vi "串口采集电压.vi"() -> ()   [LabVIEW 2018]
uses:
  <vilib>/Instr/_visa.llb/VISA Configure Serial Port (Instr).vi
panel:
  in  "波特率":u64(ring) items=["4800", "9600", "115200"]
  out "总接收":i32[][](array[numeric])
  in  "启动":bool
  in  "基路径":path
  in  "Save":bool
  out "单次接收":u8[](array[numeric])
  out "电压":string
  in  "stop bits (10: 1 bit)":u16(ring)=10 caption="停止位（10: 1位）" items=["1.0"=10, "1.5"=15, "2.0"=20]
  in  "parity (0:none)":enum16{"None", "Odd", "Even", "Mark", "Space"}(ring) caption="奇偶（0:无）"
  in  "data bits (8)":u16=8 caption="数据比特(8)" min=5 max=8 step=1
  in  "VISA resource name":refnum<visa-resource-name> caption="VISA资源名称"
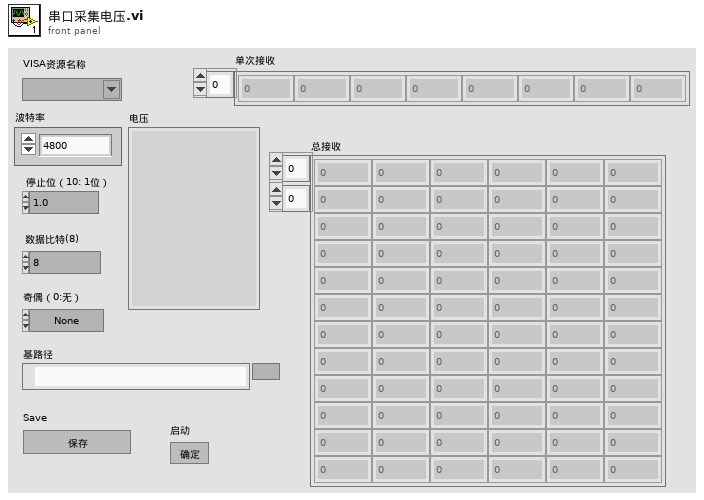
[diagram p1: front panel]
types:
  T1 = enum16{"open", "replace", "create", "open or create", "replace or create", "replace or create with confirmation"}
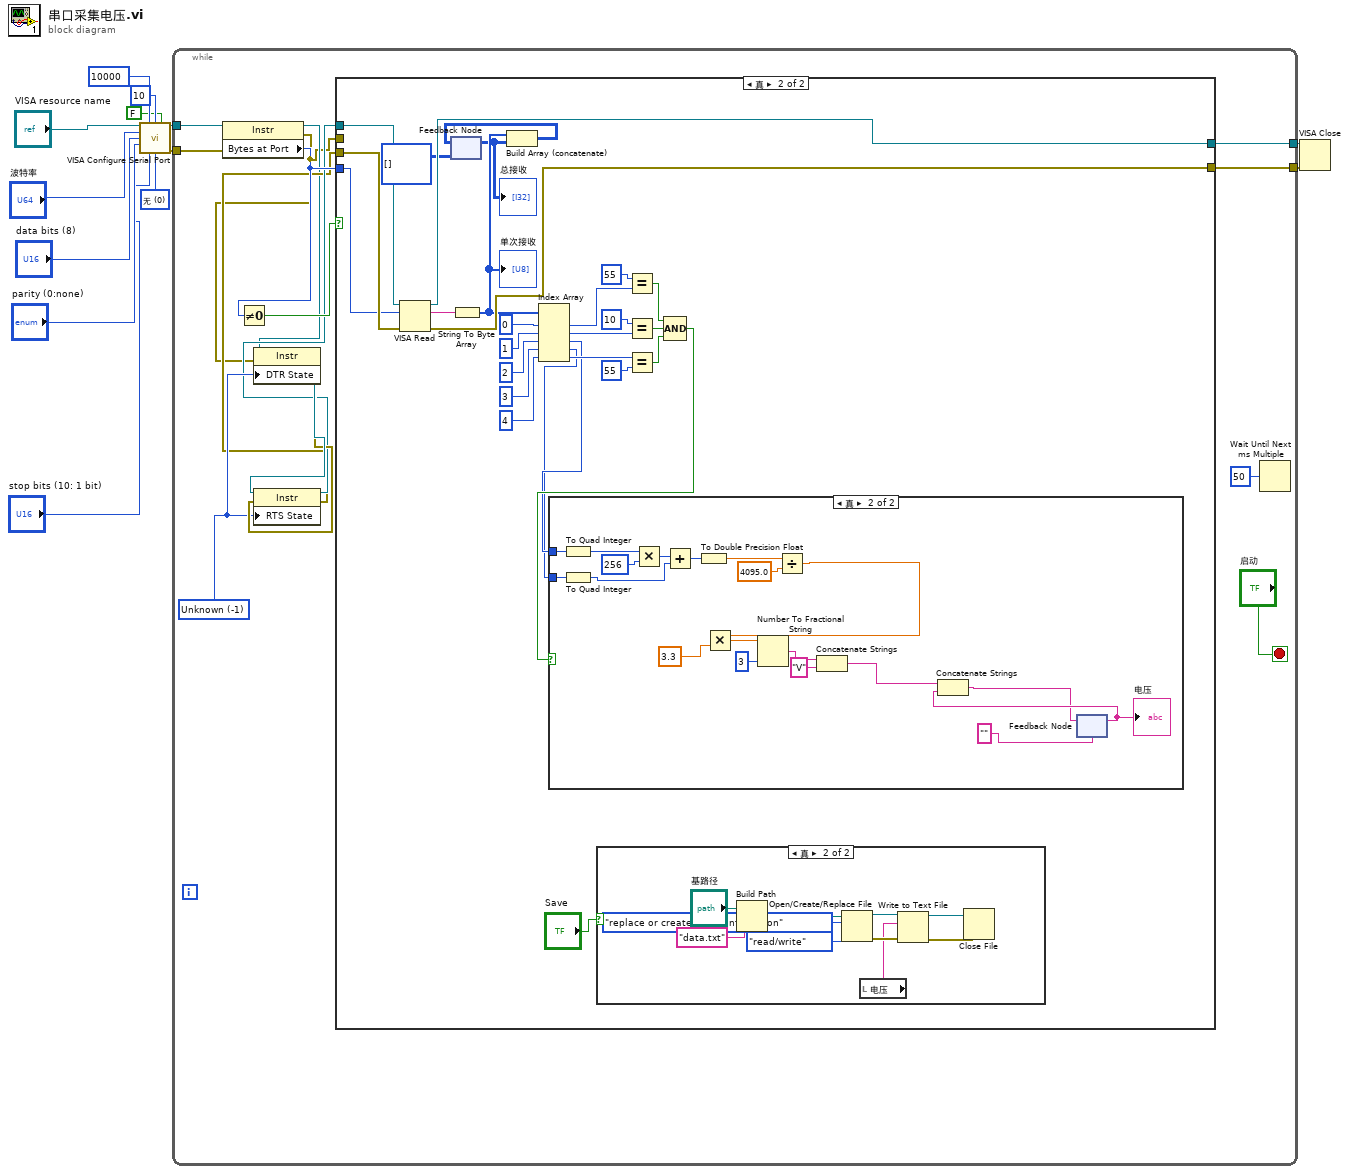
[diagram p0: block diagram]
diagram:
  w9 = u16 0 items=["无", "XON/XOFF", "RTS/CTS", "XON/XOFF & RTS/CTS", "DTR/DSR", "XON/XOFF & DTR/DSR"] ("flow control (0:none)")
  n1 = call-poly "VISA Configure Serial Port"("VISA resource name"="VISA resource name", "timeout (10sec)"=u32 10000, "termination char\n(0xA = '\\n' = LF)"=u8 10 ("termination char\n(0xA = '\\n' = LF)"), "Enable Termination\nChar (T)"=FALSE ("Enable Termination\nChar (T)"), "baud rate (9600)"="波特率", "data bits (8)"="data bits (8)", "parity (0:none)"="parity (0:none)", "stop bits (10: 1 bit)"="stop bits (10: 1 bit)", "flow control (0:none)"=w9) -> ("VISA resource name out"=w5:refnum<visa-resource-name>, "error out"=w4:errorcluster)  [unwired: 5 in]
  n2 = while {
    tunnel: w5 -> [w28]
    tunnel: w4 -> [w27]
    tunnel: [w24] -> w3
    tunnel: [w23] -> w2
    stop <- "启动" stop-if-true
    w18 = i16 -1 items=["Unknown"=-1, "Unasserted"=0, "Asserted"=1] ("Serial Settings:Modem Line Settings:Line DTR State")
    n3 = property class="Instr"(reference=w28, error in=w27) -> (reference out=w15:refnum<visa-resource-name>, error out=w14:errorcluster, "Bytes at Port"=w25:u32)
    n4 = Not Equal To 0?(x=w25) -> (x != 0?=w26:bool)
    n5 = property class="Instr"(reference=w15, error in=w14, "DTR State"=w18) -> (reference out=w20:refnum<visa-resource-name>, error out=w19:errorcluster)
    n6 = property class="Instr"(reference=w20, error in=w19, "RTS State"=w18) -> (reference out=w17:refnum<visa-resource-name>, error out=w16:errorcluster)
    n7 = case shown="真" w26 {
      tunnel: w17 -> [_ w56]
      tunnel: w16 -> [_ w55]
      tunnel: w25 -> [_ w54]
      tunnel: [_ w53] -> w24
      tunnel: [_ w52] -> w23
      tunnel: w14 -> [_ _]
      frame False {
      }
      frame True {
        n8 = VISA Read(VISA resource name=w56, byte count=w54, error in (no error)=w55) -> (VISA resource name out=w53:refnum<visa-resource-name>, read buffer=w49:string, error out=w52:errorcluster)  [unwired: 1 out]
        n9 = feedback #1(i32[][] []) -> (w44:i32[][])
        "总接收" <- w44
        n10 = String To Byte Array(string=w49) -> (unsigned byte array=w45:u8[])
        "单次接收" <- w45
        n11 = Build Array (concatenate)(w45, w44) -> (w46:i32[][])
        n12 = feedback-in #1(w46) -> ()
        n13 = Index Array(array=w45, index #1=0 ("索引"), index #2=1 ("索引"), index #3=2 ("索引"), index #4=3 ("索引"), index #5=4 ("索引")) -> (element #1=w42:u8, element #2=w40:u8, element #3=w31:u8, element #4=w30:u8, element #5=w32:u8)
        n14 = case shown="真" "Save" {
          frame False {
          }
          frame True {
            n15 = Build Path(base path="基路径", name or relative path="data.txt" ("名称或相对路径")) -> (appended path=w64:path)
            n16 = Open/Create/Replace File(file path (use dialog)=w64, operation (0:open)=T1."replace or create with confirmation" ("操作(0:open)"), access (0:read/write)=enum16{"read/write", "read-only", "write-only"}."read/write" ("权限(0:read/write)")) -> (refnum out=w61:refnum<file>, error out=w60:errorcluster)  [unwired: 3 in, 1 out]
            n17 = local read "电压"() -> (w57:string)
            n18 = Write to Text File(file (use dialog)=w61, text=w57, error in=w60) -> (refnum out=w59:refnum<file>, error out=w58:errorcluster)  [unwired: 1 in, 1 out]
            n19 = Close File(refnum=w59, error in=w58) -> ()  [unwired: 2 out]
          }
        }
        n20 = Equal?(x=u8 55, y=w42) -> (x = y?=w37:bool)
        n21 = Equal?(x=u8 10, y=w40) -> (x = y?=w36:bool)
        n22 = Equal?(x=w32, y=u8 55) -> (x = y?=w35:bool)
        n23 = Compound Arithmetic op=AND ("复合运算")(w37, w36, w35) -> (w34:bool)
        n24 = case shown="真" w34 {
          tunnel: w31 -> [_ w68]
          tunnel: w30 -> [_ w67]
          frame False {
          }
          frame True {
            n25 = To Quad Integer(1:w68) -> (0:w69:i64)
            n26 = To Quad Integer(1:w67) -> (0:w72:i64)
            n27 = Multiply(x=w69, y=i64 256) -> (x*y=w71:i64)
            n28 = Add(x=w71, y=w72) -> (x+y=w73:i64)
            n29 = To Double Precision Float(number=w73) -> (double precision float=w74:dbl)
            n30 = Divide(x=w74, y=4095.0) -> (x/y=w76:dbl)
            n31 = Multiply(x=w76, y=3.3) -> (x*y=w78:dbl)
            n32 = Number To Fractional String(number=w78, precision (6)=i16 3 ("精度(6)")) -> (F-format string=w80:string)  [unwired: 2 in]
            n33 = Concatenate Strings(w80, "V" ("字符串")) -> (w82:string)
            n34 = feedback #2("") -> (w85:string)
            "电压" <- w85
            n35 = Concatenate Strings(w82, w85) -> (w83:string)
            n36 = feedback-in #2(w83) -> ()
          }
        }
      }
    }
    n37 = Wait Until Next ms Multiple(millisecond multiple=u32 50 ("毫秒倍数")) -> ()  [unwired: 1 out]
  }
  n38 = VISA Close(VISA resource name=w3, error in (no error)=w2) -> ()  [unwired: 1 out]
